vi "WPI_MotorControlOpen.vi"   [LabVIEW 2017]
doc: "Opens a reference to the motor controller you specify. \n\nThis software is licensed. Open the labview\\readme\\WPI Robotics Library Open Source License.txt file for more information."
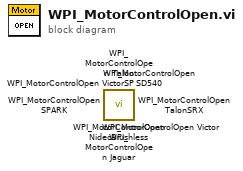
[diagram p0: block diagram]
diagram:
  n1 = call <vilib>:"WPI_MotorControlOpen NidecBrushless.vi"() -> ()  [unwired: 10 in, 2 out]
  n2 = call <vilib>:"WPI_MotorControlOpen SD540.vi"() -> ()  [unwired: 10 in, 2 out]
  n3 = call <vilib>:"WPI_MotorControlOpen SPARK.vi"() -> ()  [unwired: 10 in, 2 out]
  n4 = call <vilib>:"WPI_MotorControlOpen TalonSRX.vi"() -> ()  [unwired: 10 in, 2 out]
  n5 = call <vilib>:"WPI_MotorControlOpen VictorSP.vi"() -> ()  [unwired: 10 in, 2 out]
  n6 = call <vilib>:"WPI_MotorControlOpen Talon.vi"() -> ()  [unwired: 10 in, 2 out]
  n7 = call <vilib>:"WPI_MotorControlOpen Victor.vi"() -> ()  [unwired: 10 in, 2 out]
  n8 = call <vilib>:"WPI_MotorControlOpen Jaguar.vi"() -> ()  [unwired: 10 in, 2 out]
